vi "Handle Error.vi"(8 "error in (no error)":errorcluster, 11 "LNA_GoBang in":refnum<class "LNA_GoBang.lvclass">) -> (0 "error out":errorcluster, 2 "stop actor?":bool=TRUE, 3 "LNA_GoBang out":refnum<class "LNA_GoBang.lvclass">)   [LabVIEW 2014, in "GoBang.lvlib" / "LNA_GoBang.lvclass"]
doc: "(<B>Filename</B>: Actor Framework.lvlib:Actor.lvclass:Handle Error.vi)\n\nDefines how the actor handles an error that occurred while processing a message.\n\nBy default, this method does nothing except stop the actor. This method also treats error code 43 (coming from <B>error in</B>) as a sign that the actor shut down normally. In this situation, the Handle Error method does not return the error on <B>error out</B>, meaning the actor's caller will not receive it. All other error codes will be returned on <B>error out</B>.\n\nA descendant class may override this method to change this behavior."
uses:
  LNA_GoBang.lvclass
  <vilib>/ActorFramework/Actor/Actor.lvclass/Actor.ctl
  <vilib>/ActorFramework/Report Error Msg/Report Error Msg.lvclass/Report Error Msg.ctl
  <vilib>/ActorFramework/Message Enqueuer/Message Enqueuer.lvclass/Message Enqueuer.ctl
  <vilib>/ActorFramework/Message Enqueuer/Enqueue.vi
  <vilib>/ActorFramework/Message Priority Queue/Priority Enqueue.vi
  <vilib>/ActorFramework/Report Error Msg/Report Error Msg.lvclass
  <vilib>/NI/Actors/Linked Network Actor/Linked Network Actor/Linked Network Actor.lvclass
  <vilib>/ActorFramework/Actor/Actor.lvclass
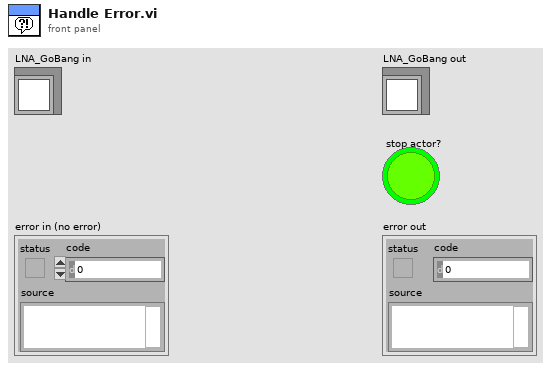
[diagram p1: front panel]
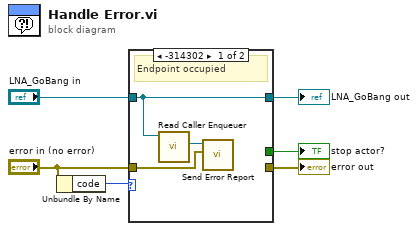
[diagram p0: block diagram]
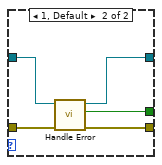
[diagram p2: hidden frame]
diagram:
  n1 = Unbundle By Name("error in (no error)") -> ("code"=w1:i32)
  n2 = case shown="-314302" w1 {
    tunnel: [_ w14] -> w6
    tunnel: [_ w13] -> w5
    tunnel: [w8 w12] -> w4
    tunnel: "error in (no error)" -> [w7 w11]
    tunnel: "LNA_GoBang in" -> [w8 w10]
    frame -314302 {
      # "Endpoint occupied"
      n3 = call <vilib>:"Read Caller Enqueuer.vi"("Actor"=w8) -> ("Caller Enqueuer"=w9:refnum<class "Message Enqueuer.lvclass">)  [unwired: 10 in]
      n4 = call <vilib>:"Send Error Report.vi"("Error From Sender"=w7, "Message Enqueuer"=w9) -> ()  [unwired: 9 in, 1 out]
    }
    frame 1, Default {
      n5 = call-parent "Handle Error.vi"("error in (no error)"=w11, "Linked Network Actor in"=w10) -> ("error out"=w14:errorcluster, "stop actor?"=w13:bool, "Linked Network Actor out"=w12:refnum<class "LNA_GoBang.lvclass">)  [unwired: 7 in]
    }
  }
  "LNA_GoBang out" <- w4
  "error out" <- w6
  "stop actor?" <- w5
